vi "Loop_SM.vi"() -> ()   [LabVIEW 2017, in "Hopper System.lvlib"]
uses:
  Hopper System.lvlib
  Cluster_CMD to SM Data.ctl
  ENUM_Firing_State.ctl
  ENUM_State.ctl
  ENUM_Action.ctl
  Globals/Global_STOP.vi
  Global_HW Status.vi
  Globals/Global_CMD to SM Data.vi
  Globals/Global_Hopper Statis.vi
  Global_SM_Data Out.vi
panel:
  out "Prefomed\nState":T1
  out "Requested\nState":T1
  out "Inner Out":dbl
  out "Inner Motor Speed":dbl=0.4
  out "Load Out":dbl
  out "Balls Shot":i32
  out "Loader Speed":dbl=0.4
  out "Hopper_CMD":T2={"Enable Loading"=FALSE, "Disable Loading"=FALSE, "Fireing State"=enum."No Fireing", "Time Limit Loading"=0.0, "Time Limit Rapid"=0.0, "Rapid Fire Shot Limit"=3, "Shotgun Fire Shot Limit"=1}
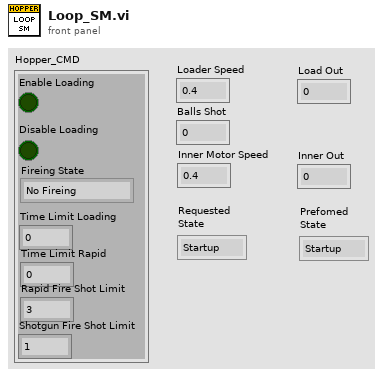
[diagram p1: front panel]
types:
  T1 = typedef "Hopper System.lvlib/ENUM_State.ctl" = enum16{"Startup", "Idle", "Loading", "Ball Ready", "Shotgun Fire", "Rapid Fire", "5 Second", "Hopper E-STOP", "Shutdown"}
  T2 = typedef "Hopper System.lvlib/Cluster_CMD to SM Data.ctl" = cluster{"Enable Loading":bool, "Disable Loading":bool, "Fireing State":T3, "Time Limit Loading":dbl, "Time Limit Rapid":dbl, "Rapid Fire Shot Limit":i32, "Shotgun Fire Shot Limit":i32}
  T3 = typedef "Hopper System.lvlib/ENUM_Firing_State.ctl" = enum16{"No Fireing", "Rapid Fire", "Shotgun Fireing"}
  T4 = typedef "Hopper System.lvlib/ENUM_Action.ctl" = enum16{"No Action", "Reset Time", "Check Time Loading", "Check Time Rapid", "Reset All", "Loader Run", "Reset Loader", "Reset Counter", "Check Counter", "Inner Motor Run", "Reset Inner Motor", "Reset Shooting", "Shooting Complete"}
  T5 = cluster{"Actions":T4[], "State":T1, "Current Time":timestamp, "Start Time":timestamp, "Loop Time (ms)":u32, "Hopper_CMD":T2, "Loader OUT":dbl, "Ball Present":bool, "Current Shots Fired":i32, "Loader Speed":dbl, "Time Limit Passed Load":bool, "Time Limit Passed Rapid":bool, "Start Shots Fired":i32, "Shotgun Fire Limit Passed":bool, "Rapid Fire Limit Passed":bool, "Inner Motor Speed":dbl, "Inner Motor Speed OUT":dbl, "Shooting Complete":bool}
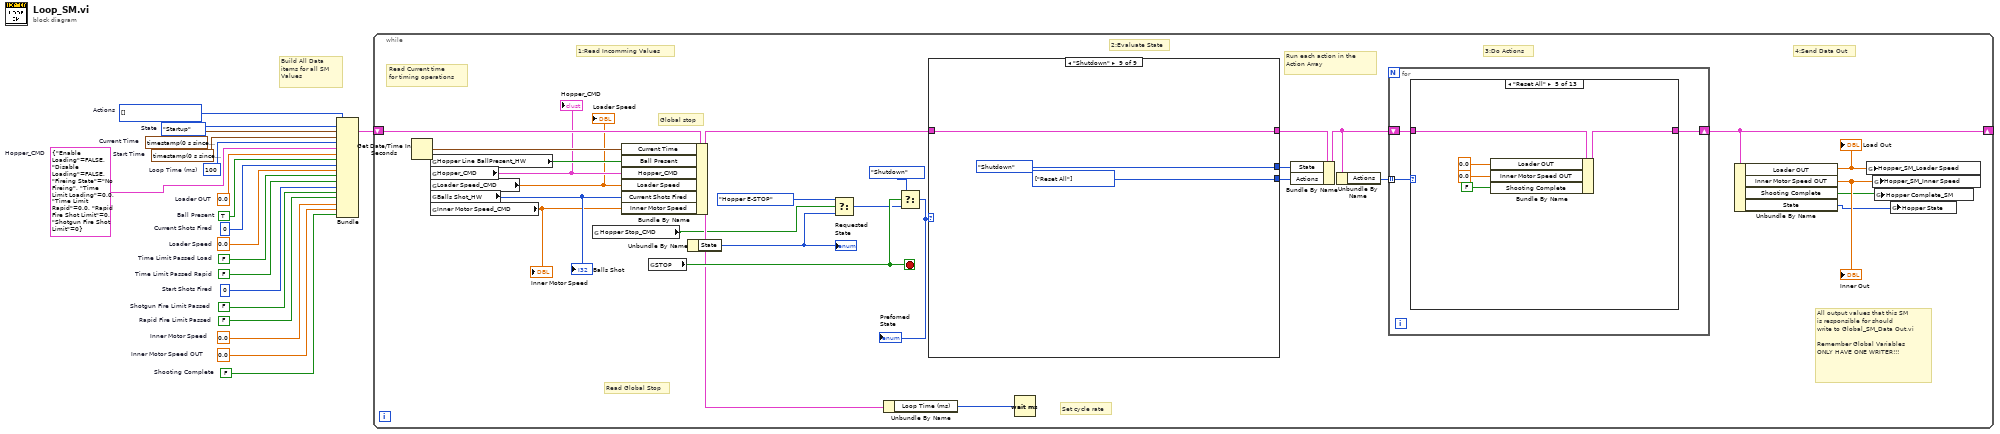
[diagram p0: block diagram]
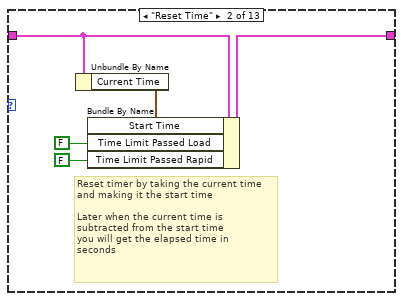
[diagram p3: hidden frame]
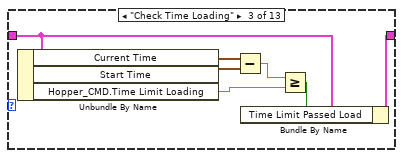
[diagram p4: hidden frame]
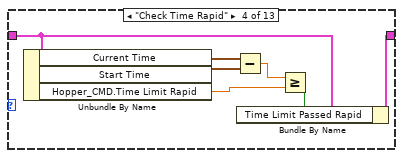
[diagram p5: hidden frame]
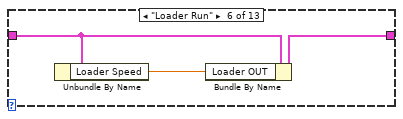
[diagram p6: hidden frame]
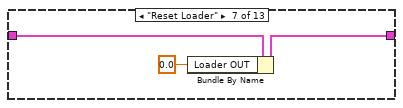
[diagram p7: hidden frame]
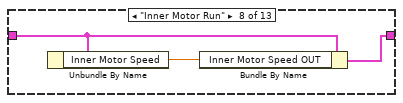
[diagram p8: hidden frame]
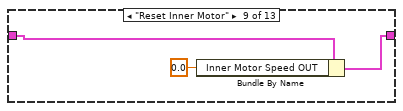
[diagram p9: hidden frame]
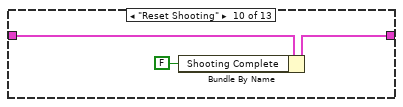
[diagram p10: hidden frame]
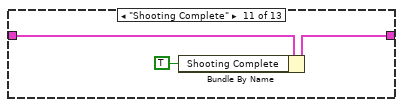
[diagram p11: hidden frame]
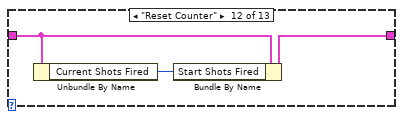
[diagram p12: hidden frame]
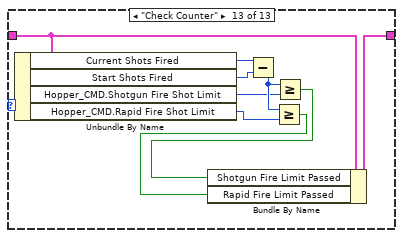
[diagram p13: hidden frame]
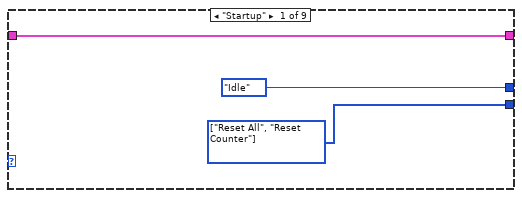
[diagram p14: hidden frame]
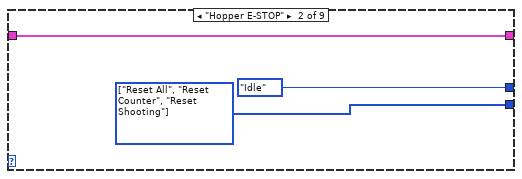
[diagram p15: hidden frame]
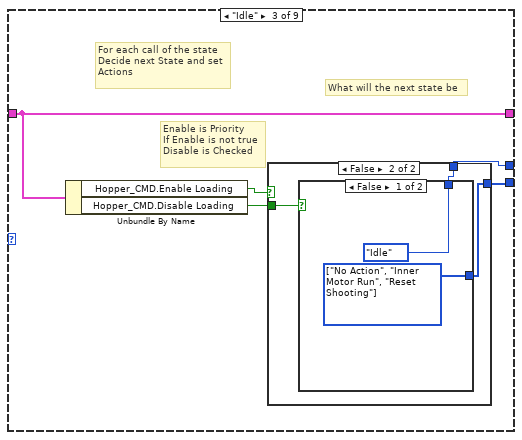
[diagram p16: hidden frame]
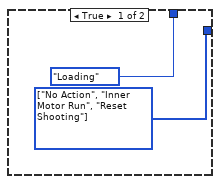
[diagram p17: hidden frame]
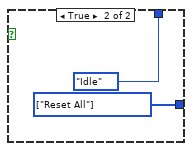
[diagram p18: hidden frame]
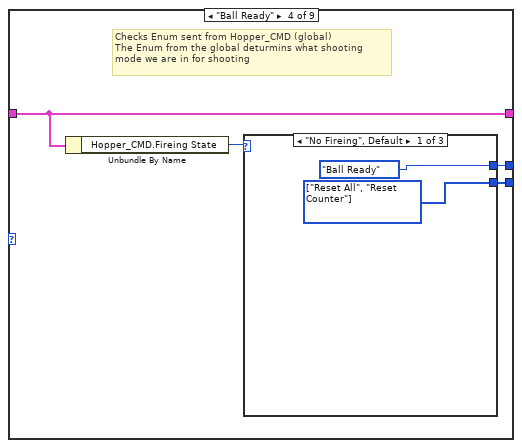
[diagram p19: hidden frame]
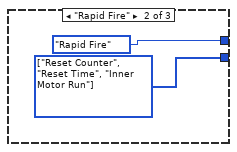
[diagram p20: hidden frame]
diagram:
  w1 = FALSE  # Shooting Complete
  w2 = 0.0  # Inner Motor Speed OUT
  w3 = 0.0  # Inner Motor Speed
  w4 = FALSE  # Rapid Fire Limit Passed
  w5 = FALSE  # Shotgun Fire Limit Passed
  w6 = 0  # Start Shots Fired
  w7 = FALSE  # Time Limit Passed Rapid
  w8 = FALSE  # Time Limit Passed Load
  w9 = 0.0  # Loader Speed
  w10 = 0  # Current Shots Fired
  w11 = T2 {"Enable Loading"=FALSE, "Disable Loading"=FALSE, "Fireing State"=enum."No Fireing", "Time Limit Loading"=0.0, "Time Limit Rapid"=0.0, "Rapid Fire Shot Limit"=0, "Shotgun Fire Shot Limit"=0}  # Hopper_CMD
  w12 = TRUE  # Ball Present
  w13 = u32 100  # Loop Time (ms)
  w14 = T4[] [] items=["No Action", "Reset Time", "Check Time Loading", "Check Time Rapid", "Reset All", "Loader Run", "Reset Loader", "Reset Counter", "Check Counter", "Inner Motor Run", "Reset Inner Motor", "Reset Shooting", "Shooting Complete"]  # Actions
  w15 = 0.0  # Loader OUT
  w16 = timestamp(0 s since 1904-01-01)  # Start Time
  w17 = timestamp(0 s since 1904-01-01)  # Current Time
  w18 = ENUM_State."Startup"  # State
  # "Build All Data items for all SM Values"
  n1 = Bundle("Actions"=w14, "State"=w18, "Current Time"=w17, "Start Time"=w16, "Loop Time (ms)"=w13, "Hopper_CMD"=w11, "Loader OUT"=w15, "Ball Present"=w12, "Current Shots Fired"=w10, "Loader Speed"=w9, "Time Limit Passed Load"=w8, "Time Limit Passed Rapid"=w7, "Start Shots Fired"=w6, "Shotgun Fire Limit Passed"=w5, "Rapid Fire Limit Passed"=w4, "Inner Motor Speed"=w3, "Inner Motor Speed OUT"=w2, "Shooting Complete"=w1) -> (w19:T5)  [unwired: 1 in]
  n2 = while {
    shift-right: [w35] -> _
    shift-left: w19 -> [w44]
    stop <- w38 stop-if-true
    # "Set cycle rate"
    # "All output values that this SM\nis responsible for should\nwrite to Global_SM_Data Out.vi\n\nRemember Global Variables\nONLY HAVE ONE WRITER!!!"
    # "Read Current time\nfor timing operations"
    # "Run each action in the Action Array"
    # "Read Global Stop"
    # "1:Read Incomming Values"
    # "2:Evaluate State"
    # "3:Do Actions"
    # "4:Send Data Out"
    # "Global stop"
    n3 = Get Date/Time In Seconds() -> (seconds since 1Jan1904=w43:timestamp)
    n4 = global read "Global_HW Status.vi" "Hopper Line BallPresent_HW"() -> (w31:bool)
    n5 = global read "Global_CMD to SM Data.vi" "Hopper_CMD"() -> (w30:T2)
    "Hopper_CMD" <- w30
    n6 = global read "Global_CMD to SM Data.vi" "Loader Speed_CMD"() -> (w25:dbl)
    "Loader Speed" <- w25
    n7 = global read "Global_HW Status.vi" "Balls Shot_HW"() -> (w29:i32)
    "Balls Shot" <- w29
    n8 = global read "Global_CMD to SM Data.vi" "Inner Motor Speed_CMD"() -> (w24:dbl)
    "Inner Motor Speed" <- w24
    n9 = global read "Global_CMD to SM Data.vi" "Hopper Stop_CMD"() -> (w23:bool)
    n10 = Bundle By Name(cluster=w44, "Current Time"=w43, "Ball Present"=w31, "Hopper_CMD"=w30, "Loader Speed"=w25, "Current Shots Fired"=w29, "Inner Motor Speed"=w24) -> (w33:T5)
    n11 = global read "Global_STOP.vi" "STOP"() -> (w38:bool)
    n12 = Unbundle By Name(w33) -> ("State"=w27:T1)
    "Requested\nState" <- w27
    n13 = Select(t=ENUM_State."Hopper E-STOP" ("State"), s=w23, f=w27) -> (s? t:f=w28:T1)
    n14 = Unbundle By Name(w33) -> ("Loop Time (ms)"=w34:u32)
    n15 = Select(t=ENUM_State."Shutdown" ("State"), s=w38, f=w28) -> (s? t:f=w36:T1)
    "Prefomed\nState" <- w36
    n16 = case shown="\"Shutdown\"" w36 {
      tunnel: w33 -> [w106 w109 w114 w127 w137 w146 w160 w175 w193]
      tunnel: [w106 w109 w114 w127 w137 w146 w160 w175 w193] -> w41
      tunnel: [ENUM_State."Idle" ("State") ENUM_State."Idle" ("State") w112 w125 w135 w144 w159 w174 ENUM_State."Shutdown" ("State")] -> w40
      tunnel: [w105 w107 w111 w124 w136 w145 w158 w173 w191] -> w39
      frame "Startup" {
        w105 = T4[] [enum."Reset All", enum."Reset Counter"] items=["No Action", "Reset Time", "Check Time Loading", "Check Time Rapid", "Reset All", "Loader Run", "Reset Loader", "Reset Counter", "Check Counter", "Inner Motor Run", "Reset Inner Motor", "Reset Shooting", "Shooting Complete"] ("Actions")
      }
      frame "Hopper E-STOP" {
        w107 = T4[] [enum."Reset All", enum."Reset Counter", enum."Reset Shooting"] items=["No Action", "Reset Time", "Check Time Loading", "Check Time Rapid", "Reset All", "Loader Run", "Reset Loader", "Reset Counter", "Check Counter", "Inner Motor Run", "Reset Inner Motor", "Reset Shooting", "Shooting Complete"] ("Actions")
      }
      frame "Idle" {
        # "Enable is Priority\nIf Enable is not true\nDisable is Checked"
        # "For each call of the state\nDecide next State and set\nActions"
        # "What will the next state be"
        n17 = Unbundle By Name(w114) -> ("Hopper_CMD.Enable Loading"=w113:bool, "Hopper_CMD.Disable Loading"=w110:bool)
        n18 = case shown="False" w113 {
          tunnel: [ENUM_State."Loading" ("State") w118] -> w112
          tunnel: [w115 w117] -> w111
          tunnel: w110 -> [_ w119]
          frame True {
            w115 = T4[] [enum."No Action", enum."Inner Motor Run", enum."Reset Shooting"] items=["No Action", "Reset Time", "Check Time Loading", "Check Time Rapid", "Reset All", "Loader Run", "Reset Loader", "Reset Counter", "Check Counter", "Inner Motor Run", "Reset Inner Motor", "Reset Shooting", "Shooting Complete"] ("Actions")
          }
          frame False {
            n19 = case shown="False" w119 {
              tunnel: [ENUM_State."Idle" ("State") ENUM_State."Idle" ("State")] -> w118
              tunnel: [w120 w122] -> w117
              frame False {
                w120 = T4[] [enum."No Action", enum."Inner Motor Run", enum."Reset Shooting"] items=["No Action", "Reset Time", "Check Time Loading", "Check Time Rapid", "Reset All", "Loader Run", "Reset Loader", "Reset Counter", "Check Counter", "Inner Motor Run", "Reset Inner Motor", "Reset Shooting", "Shooting Complete"] ("Actions")
              }
              frame True {
                w122 = T4[] [enum."Reset All"] items=["No Action", "Reset Time", "Check Time Loading", "Check Time Rapid", "Reset All", "Loader Run", "Reset Loader", "Reset Counter", "Check Counter", "Inner Motor Run", "Reset Inner Motor", "Reset Shooting", "Shooting Complete"] ("Actions")
              }
            }
          }
        }
      }
      frame "Ball Ready" {
        # "Checks Enum sent from Hopper_CMD (global)\nThe Enum from the global deturmins what shooting\nmode we are in for shooting"
        n20 = Unbundle By Name(w127) -> ("Hopper_CMD.Fireing State"=w126:T3)
        n21 = case shown="\"No Fireing\", Default" w126 {
          tunnel: [ENUM_State."Ball Ready" ("State") ENUM_State."Rapid Fire" ("State") ENUM_State."Shotgun Fire" ("State")] -> w125
          tunnel: [w128 w130 w132] -> w124
          frame "No Fireing", Default {
            w128 = T4[] [enum."Reset All", enum."Reset Counter"] items=["No Action", "Reset Time", "Check Time Loading", "Check Time Rapid", "Reset All", "Loader Run", "Reset Loader", "Reset Counter", "Check Counter", "Inner Motor Run", "Reset Inner Motor", "Reset Shooting", "Shooting Complete"] ("Actions")
          }
          frame "Rapid Fire" {
            w130 = T4[] [enum."Reset Counter", enum."Reset Time", enum."Inner Motor Run"] items=["No Action", "Reset Time", "Check Time Loading", "Check Time Rapid", "Reset All", "Loader Run", "Reset Loader", "Reset Counter", "Check Counter", "Inner Motor Run", "Reset Inner Motor", "Reset Shooting", "Shooting Complete"] ("Actions")
          }
          frame "Shotgun Fireing" {
            w132 = T4[] [enum."Reset Counter", enum."Inner Motor Run", enum."Reset Shooting"] items=["No Action", "Reset Time", "Check Time Loading", "Check Time Rapid", "Reset All", "Loader Run", "Reset Loader", "Reset Counter", "Check Counter", "Inner Motor Run", "Reset Inner Motor", "Reset Shooting", "Shooting Complete"] ("Actions")
          }
        }
      }
      frame "Shotgun Fire" {
        n22 = Unbundle By Name(w137) -> ("Shotgun Fire Limit Passed"=w134:bool)
        n23 = case shown="True" w134 {
          tunnel: [w138 w141] -> w136
          tunnel: [ENUM_State."Shotgun Fire" ("State") ENUM_State."Loading" ("State")] -> w135
          frame False {
            w138 = T4[] [enum."Loader Run", enum."Check Counter", enum."Inner Motor Run", enum."Reset Shooting"] items=["No Action", "Reset Time", "Check Time Loading", "Check Time Rapid", "Reset All", "Loader Run", "Reset Loader", "Reset Counter", "Check Counter", "Inner Motor Run", "Reset Inner Motor", "Reset Shooting", "Shooting Complete"] ("Actions")
          }
          frame True {
            w141 = T4[] [enum."Reset All", enum."Reset Counter", enum."Shooting Complete"] items=["No Action", "Reset Time", "Check Time Loading", "Check Time Rapid", "Reset All", "Loader Run", "Reset Loader", "Reset Counter", "Check Counter", "Inner Motor Run", "Reset Inner Motor", "Reset Shooting", "Shooting Complete"] ("Actions")
          }
        }
      }
      frame "Rapid Fire" {
        n24 = Unbundle By Name(w146) -> ("Time Limit Passed Rapid"=w143:bool, "Rapid Fire Limit Passed"=w142:bool)
        n25 = case shown="True" w143 {
          tunnel: w142 -> [_ w151]
          tunnel: [w147 w150] -> w145
          tunnel: [ENUM_State."Loading" ("State") w149] -> w144
          frame True {
            w147 = T4[] [enum."Inner Motor Run", enum."Reset Time", enum."Reset Counter", enum."Shooting Complete"] items=["No Action", "Reset Time", "Check Time Loading", "Check Time Rapid", "Reset All", "Loader Run", "Reset Loader", "Reset Counter", "Check Counter", "Inner Motor Run", "Reset Inner Motor", "Reset Shooting", "Shooting Complete"] ("Actions")
          }
          frame False {
            n26 = case shown="False" w151 {
              tunnel: [w153 w155] -> w150
              tunnel: [ENUM_State."Loading" ("State") ENUM_State."Rapid Fire" ("State")] -> w149
              frame True {
                w153 = T4[] [enum."Reset All", enum."Reset Time", enum."Reset Counter", enum."Shooting Complete"] items=["No Action", "Reset Time", "Check Time Loading", "Check Time Rapid", "Reset All", "Loader Run", "Reset Loader", "Reset Counter", "Check Counter", "Inner Motor Run", "Reset Inner Motor", "Reset Shooting", "Shooting Complete"] ("Actions")
              }
              frame False {
                w155 = T4[] [enum."Loader Run", enum."Check Time Rapid", enum."Check Counter", enum."Inner Motor Run", enum."Reset Shooting"] items=["No Action", "Reset Time", "Check Time Loading", "Check Time Rapid", "Reset All", "Loader Run", "Reset Loader", "Reset Counter", "Check Counter", "Inner Motor Run", "Reset Inner Motor", "Reset Shooting", "Shooting Complete"] ("Actions")
              }
            }
          }
        }
      }
      frame "Loading" {
        n27 = Unbundle By Name(w160) -> ("Ball Present"=w156:bool, "Hopper_CMD.Disable Loading"=w157:bool)
        n28 = case shown="False" w157 {
          tunnel: [ENUM_State."Idle" ("State") w165] -> w159
          tunnel: [w162 w164] -> w158
          tunnel: w156 -> [_ w163]
          frame True {
            w162 = T4[] [enum."Reset All"] items=["No Action", "Reset Time", "Check Time Loading", "Check Time Rapid", "Reset All", "Loader Run", "Reset Loader", "Reset Counter", "Check Counter", "Inner Motor Run", "Reset Inner Motor", "Reset Shooting", "Shooting Complete"] ("Actions")
          }
          frame False {
            n29 = case shown="True" w163 {
              tunnel: [ENUM_State."Ball Ready" ("State") ENUM_State."5 Second" ("State")] -> w165
              tunnel: [w166 w168] -> w164
              frame True {
                w166 = T4[] [enum."Reset Time", enum."Reset All"] items=["No Action", "Reset Time", "Check Time Loading", "Check Time Rapid", "Reset All", "Loader Run", "Reset Loader", "Reset Counter", "Check Counter", "Inner Motor Run", "Reset Inner Motor", "Reset Shooting", "Shooting Complete"] ("Actions")
              }
              frame False {
                w168 = T4[] [enum."Reset Time", enum."Loader Run", enum."Inner Motor Run"] items=["No Action", "Reset Time", "Check Time Loading", "Check Time Rapid", "Reset All", "Loader Run", "Reset Loader", "Reset Counter", "Check Counter", "Inner Motor Run", "Reset Inner Motor", "Reset Shooting", "Shooting Complete"] ("Actions")
              }
            }
          }
        }
      }
      frame "5 Second" {
        n30 = Unbundle By Name(w175) -> ("Ball Present"=w171:bool, "Hopper_CMD.Disable Loading"=w172:bool, "Time Limit Passed Load"=w170:bool)
        n31 = case shown="True" w172 {
          tunnel: [ENUM_State."Idle" ("State") w181] -> w174
          tunnel: [w177 w180] -> w173
          tunnel: w171 -> [_ w179]
          tunnel: w170 -> [_ w178]
          frame True {
            w177 = T4[] [enum."Reset All"] items=["No Action", "Reset Time", "Check Time Loading", "Check Time Rapid", "Reset All", "Loader Run", "Reset Loader", "Reset Counter", "Check Counter", "Inner Motor Run", "Reset Inner Motor", "Reset Shooting", "Shooting Complete"] ("Actions")
          }
          frame False {
            n32 = case shown="True" w179 {
              tunnel: [ENUM_State."Loading" ("State") w186] -> w181
              tunnel: [w182 w185] -> w180
              tunnel: w178 -> [_ w184]
              frame True {
                w182 = T4[] [enum."Reset All"] items=["No Action", "Reset Time", "Check Time Loading", "Check Time Rapid", "Reset All", "Loader Run", "Reset Loader", "Reset Counter", "Check Counter", "Inner Motor Run", "Reset Inner Motor", "Reset Shooting", "Shooting Complete"] ("Actions")
              }
              frame False {
                n33 = case shown="True" w184 {
                  tunnel: [ENUM_State."Idle" ("State") ENUM_State."5 Second" ("State")] -> w186
                  tunnel: [w187 w189] -> w185
                  frame True {
                    w187 = T4[] [enum."Reset Time", enum."Reset All"] items=["No Action", "Reset Time", "Check Time Loading", "Check Time Rapid", "Reset All", "Loader Run", "Reset Loader", "Reset Counter", "Check Counter", "Inner Motor Run", "Reset Inner Motor", "Reset Shooting", "Shooting Complete"] ("Actions")
                  }
                  frame False {
                    w189 = T4[] [enum."Check Time Loading", enum."Loader Run", enum."Inner Motor Run", enum."Reset Shooting"] items=["No Action", "Reset Time", "Check Time Loading", "Check Time Rapid", "Reset All", "Loader Run", "Reset Loader", "Reset Counter", "Check Counter", "Inner Motor Run", "Reset Inner Motor", "Reset Shooting", "Shooting Complete"] ("Actions")
                  }
                }
              }
            }
          }
        }
      }
      frame "Shutdown" {
        w191 = T4[] [enum."Reset All"] items=["No Action", "Reset Time", "Check Time Loading", "Check Time Rapid", "Reset All", "Loader Run", "Reset Loader", "Reset Counter", "Check Counter", "Inner Motor Run", "Reset Inner Motor", "Reset Shooting", "Shooting Complete"] ("Actions")
      }
    }
    n34 = Wait (ms)(milliseconds to wait=w34) -> ()  [unwired: 1 out]
    n35 = Bundle By Name(cluster=w41, "State"=w40, "Actions"=w39) -> (w42:T5)
    n36 = Unbundle By Name(w42) -> ("Actions"=w45:T4[])
    n37 = for {
      tunnel: w45 -> [w48] mode=indexing
      shift-right: [w47] -> w35
      shift-left: w42 -> [w46]
      n38 = case shown="\"Reset All\"" w48 {
        tunnel: w46 -> [w49 w54 w56 w63 w73 w75 w79 w82 w85 w88 w91 w93 w103]
        tunnel: [w49 w53 w55 w62 w72 w76 w78 w81 w84 w87 w90 w94 w102] -> w47
        frame "No Action" {
        }
        frame "Reset Time" {
          # "Reset timer by taking the current time\nand making it the start time\n\nLater when the current time is \nsubtracted from the start time\nyou will get the elapsed time in \nseconds"
          n39 = Unbundle By Name(w54) -> ("Current Time"=w52:timestamp)
          n40 = Bundle By Name(cluster=w54, "Start Time"=w52, "Time Limit Passed Load"=FALSE, "Time Limit Passed Rapid"=FALSE) -> (w53:T5)
        }
        frame "Check Time Loading" {
          n41 = Unbundle By Name(w56) -> ("Current Time"=w61:timestamp, "Start Time"=w60:timestamp, "Hopper_CMD.Time Limit Loading"=w58:dbl)
          n42 = Subtract(x=w61, y=w60) -> (x-y=w59:dbl)
          n43 = Greater Or Equal?(x=w59, y=w58) -> (x >= y?=w57:bool)
          n44 = Bundle By Name(cluster=w56, "Time Limit Passed Load"=w57) -> (w55:T5)
        }
        frame "Check Time Rapid" {
          n45 = Unbundle By Name(w63) -> ("Current Time"=w68:timestamp, "Start Time"=w67:timestamp, "Hopper_CMD.Time Limit Rapid"=w65:dbl)
          n46 = Subtract(x=w68, y=w67) -> (x-y=w66:dbl)
          n47 = Greater Or Equal?(x=w66, y=w65) -> (x >= y?=w64:bool)
          n48 = Bundle By Name(cluster=w63, "Time Limit Passed Rapid"=w64) -> (w62:T5)
        }
        frame "Reset All" {
          n49 = Bundle By Name(cluster=w73, "Loader OUT"=0.0 ("FG Write Value"), "Inner Motor Speed OUT"=0.0, "Shooting Complete"=FALSE) -> (w72:T5)
        }
        frame "Loader Run" {
          n50 = Unbundle By Name(w75) -> ("Loader Speed"=w74:dbl)
          n51 = Bundle By Name(cluster=w75, "Loader OUT"=w74) -> (w76:T5)
        }
        frame "Reset Loader" {
          n52 = Bundle By Name(cluster=w79, "Loader OUT"=0.0 ("Percent VBus")) -> (w78:T5)
        }
        frame "Inner Motor Run" {
          n53 = Unbundle By Name(w82) -> ("Inner Motor Speed"=w80:dbl)
          n54 = Bundle By Name(cluster=w82, "Inner Motor Speed OUT"=w80) -> (w81:T5)
        }
        frame "Reset Inner Motor" {
          n55 = Bundle By Name(cluster=w85, "Inner Motor Speed OUT"=0.0) -> (w84:T5)
        }
        frame "Reset Shooting" {
          n56 = Bundle By Name(cluster=w88, "Shooting Complete"=FALSE) -> (w87:T5)
        }
        frame "Shooting Complete" {
          n57 = Bundle By Name(cluster=w91, "Shooting Complete"=TRUE) -> (w90:T5)
        }
        frame "Reset Counter" {
          n58 = Unbundle By Name(w93) -> ("Current Shots Fired"=w92:i32)
          n59 = Bundle By Name(cluster=w93, "Start Shots Fired"=w92) -> (w94:T5)
        }
        frame "Check Counter" {
          n60 = Unbundle By Name(w103) -> ("Current Shots Fired"=w101:i32, "Start Shots Fired"=w100:i32, "Hopper_CMD.Shotgun Fire Shot Limit"=w98:i32, "Hopper_CMD.Rapid Fire Shot Limit"=w97:i32)
          n61 = Subtract(x=w101, y=w100) -> (x-y=w99:i32)
          n62 = Greater Or Equal?(x=w99, y=w97) -> (x >= y?=w95:bool)
          n63 = Greater Or Equal?(x=w99, y=w98) -> (x >= y?=w96:bool)
          n64 = Bundle By Name(cluster=w103, "Shotgun Fire Limit Passed"=w96, "Rapid Fire Limit Passed"=w95) -> (w102:T5)
        }
      }
    }
    n65 = Unbundle By Name(w35) -> ("Loader OUT"=w32:dbl, "Inner Motor Speed OUT"=w22:dbl, "Shooting Complete"=w21:bool, "State"=w20:T1)
    "Load Out" <- w32
    "Inner Out" <- w22
    n66 = global write "Global_SM_Data Out.vi" "Hopper_SM_Loader Speed"(w32) -> ()
    n67 = global write "Global_SM_Data Out.vi" "Hopper_SM_Inner Speed"(w22) -> ()
    n68 = global write "Global_Hopper Statis.vi" "Hopper Complete_SM"(w21) -> ()
    n69 = global write "Global_Hopper Statis.vi" "Hopper State"(w20) -> ()
  }
